vi "initiate.vi"(8 "error in (no error)":errorcluster, 11 "reference in":refnum<class "Items Controller.lvclass">) -> (0 "error out":errorcluster, 3 "reference out":refnum<class "Items Controller.lvclass">)   [LabVIEW 2014, in "Items Controller.lvclass"]
uses:
  Items Controller.lvclass
  File Controller_llb/File Controller.lvclass
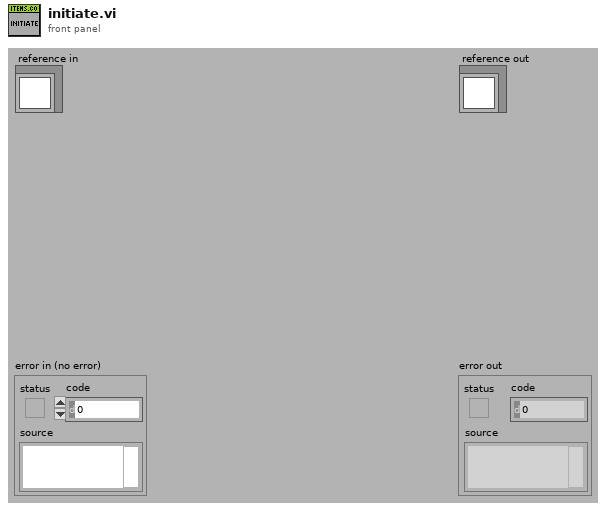
[diagram p1: front panel]
types:
  T1 = typedef "Items Controller.lvclass/ObjectAttributesRef.ctl" = refnum<data-value>
  T2 = typedef "Items Controller.lvclass/ObjectAttributes.ctl" = cluster{"MyAttribute":dbl, "data":string[][][], "file_controller_ref":refnum<class "File Controller.lvclass">, "checkIN_ref":refnum<class "checkIN.lvclass">, "checkOUT_ref":refnum<class "checkOUT.lvclass">, "item_ref":refnum<class "item.lvclass">}
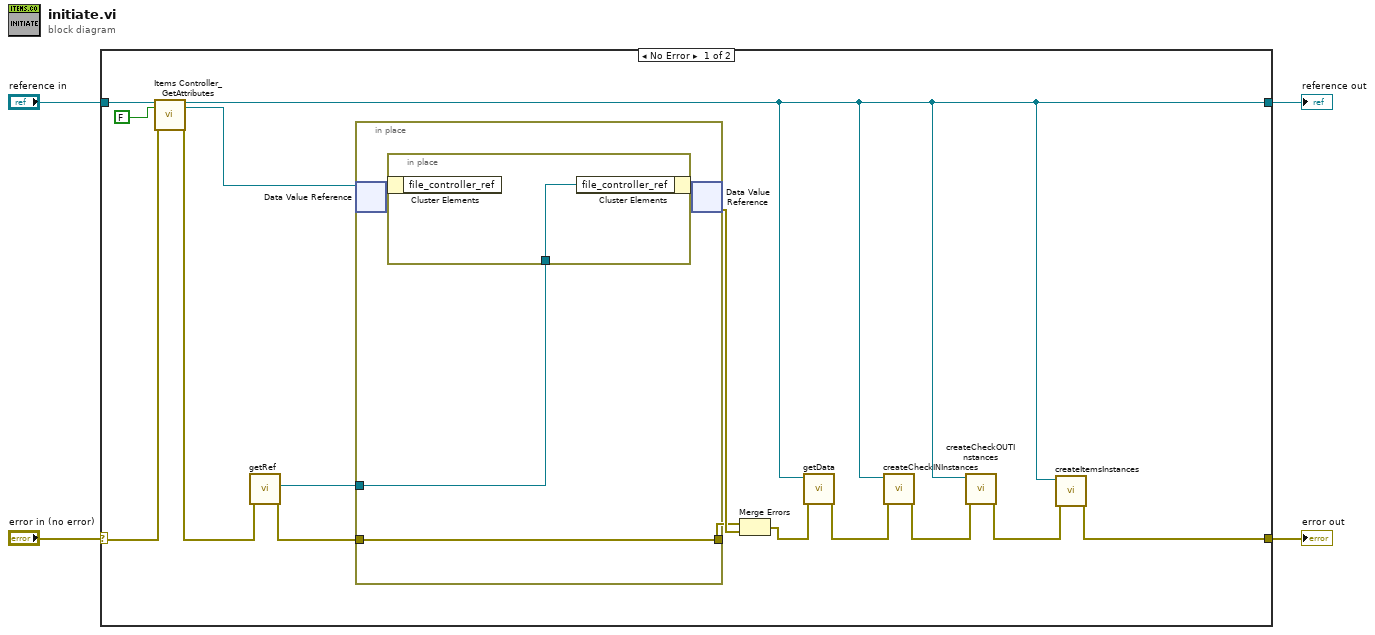
[diagram p0: block diagram]
diagram:
  n1 = case shown="No Error" "error in (no error)" {
    selector: "error in (no error)" -> [w15 w26]
    tunnel: [w5 w26] -> w3
    tunnel: [w9 w25] -> w1
    tunnel: "reference in" -> [w17 w25]
    frame No Error {
      n2 = call "Items Controller_GetAttributes.vi"("reference in"=w17, "return data? (T)"=FALSE, "error in (no error)"=w15) -> ("reference out"=w9:refnum<class "Items Controller.lvclass">, "attributes ref"=w14:T1, "error out"=w8:errorcluster)  [unwired: 13 in, 1 out]
      n3 = call "getRef.vi"("error in (no error)"=w8) -> ("error out"=w7:errorcluster, "File Controller_ref"=w6:refnum<class "File Controller.lvclass">)  [unwired: 9 in]
      n4 = in-place {
        in-place-border: w7 -> [w21]
        in-place-border: [w21] -> w18
        in-place-border: w6 -> [w20]
        n5 = in-place-dvr #1(w14) -> (w22:T2)  [unwired: 1 out]
        n6 = in-place {
          in-place-border: w20 -> [w24]
          n7 = in-place-cluster #2(w22) -> ()  [unwired: 1 out]
          n8 = in-place-cluster #2("file_controller_ref"=w24) -> (w23:T2)
        }
        n9 = in-place-dvr #1(w23) -> (w19:errorcluster)  [unwired: 1 out]
      }
      n10 = Merge Errors(w18, w19) -> (w13:errorcluster)
      n11 = call "getData.vi"("error in (no error)"=w13, "reference in"=w9) -> ("error out"=w12:errorcluster)  [unwired: 8 in, 1 out]
      n12 = call "createCheckINInstances.vi"("error in (no error)"=w12, "reference in"=w9) -> ("error out"=w11:errorcluster)  [unwired: 8 in, 1 out]
      n13 = call "createCheckOUTInstances.vi"("error in (no error)"=w11, "reference in"=w9) -> ("error out"=w10:errorcluster)  [unwired: 8 in, 1 out]
      n14 = call "createItemsInstances.vi"("error in (no error)"=w10, "reference in"=w9) -> ("error out"=w5:errorcluster)  [unwired: 8 in, 1 out]
    }
    frame Error {
    }
  }
  "error out" <- w3
  "reference out" <- w1
